vi "Create Cp plot.vi"(0 "Pressures in (cols = sensor, rows = time)":sgl[][](array[numeric])) -> (1 "Cp against x/c":cluster{"x/c flap (sorted)":sgl[], sgl[]}[](graph), 2 "Pdyn ref (Pa)":sgl)   [LabVIEW 2015]
panel:
  in  "Sensor index (sorted), cylinder":i32[](array[numeric])=[0, 1, 2, 3, 4, 5, 6, 7, 8, 9, 10, 11, 12, 13, 14, 15, 16, 17, 18, 19]
  in  "Pdyn ref sensor no.":i32=32
  in  "x/c cylinder (sorted)":sgl[](array[numeric])=[0.9659258, 0.8660254, 0.70710677, 0.5, 0.25881904, -0.25881904, -0.5, -0.70710677, -0.8660254, -0.9659258, -0.9659258, -0.8660254, -0.70710677, -0.5, -0.25881904, 0.25881904, 0.5, 0.70710677, 0.8660254, 0.9659258]
  # "Manually input and make default"
  # "Data sorted by winding no."
  # "Manually paste in data and then make default values"
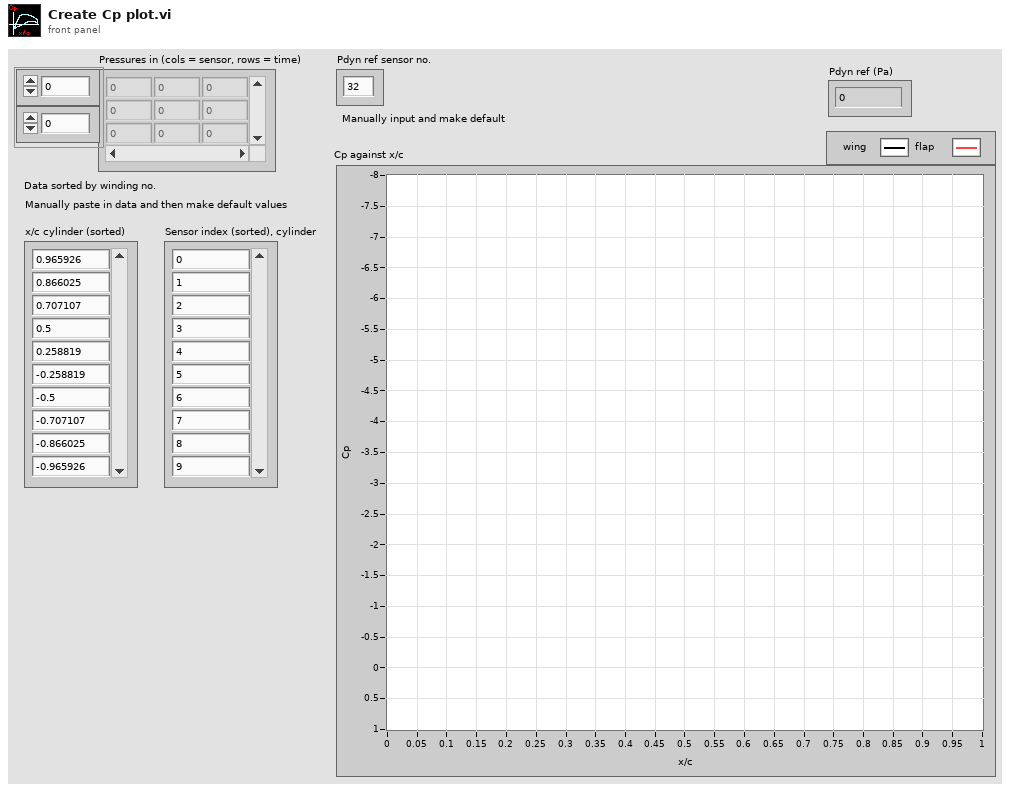
[diagram p1: front panel]
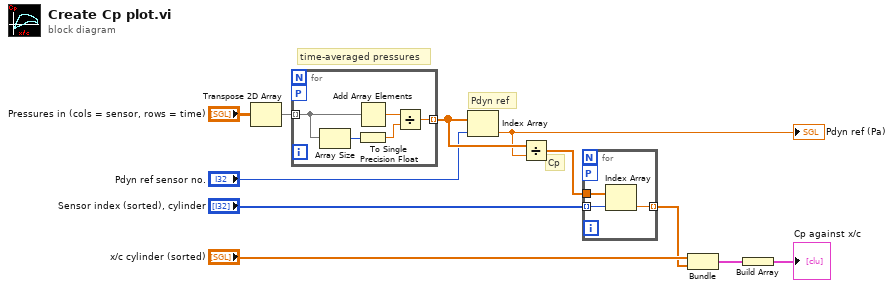
[diagram p0: block diagram]
diagram:
  # "Cp"
  # "Pdyn ref"
  # "time-averaged pressures"
  n1 = Transpose 2D Array(2D array="Pressures in (cols = sensor, rows = time)") -> (transposed array=w5:sgl[][])
  n2 = for {
    tunnel: w5 -> [w16] mode=indexing
    tunnel: [w12] -> w10 mode=indexing
    workers-P: _ -> [_]
    n3 = Array Size(array=w16) -> (size(s)=w14:i32)
    n4 = Add Array Elements(numeric array=w16) -> (sum=w15:sgl)
    n5 = To Single Precision Float(number=w14) -> (single precision float=w13:sgl)
    n6 = Divide(x=w15, y=w13) -> (x/y=w12:sgl)
  }
  n7 = Index Array(array=w10, index="Pdyn ref sensor no.") -> (element=w9:sgl)
  "Pdyn ref (Pa)" <- w9
  n8 = Divide(x=w10, y=w9) -> (x/y=w1:sgl[])
  n9 = for {
    tunnel: w1 -> [w19]
    tunnel: "Sensor index (sorted), cylinder" -> [w18] mode=indexing
    tunnel: [w17] -> w2 mode=indexing
    workers-P: _ -> [_]
    n10 = Index Array(array=w19, index=w18) -> (element=w17:sgl)
  }
  n11 = Bundle("x/c cylinder (sorted)"="x/c cylinder (sorted)", w2) -> (w6:cluster{"x/c cylinder (sorted)":sgl[], sgl[]})  [unwired: 1 in]
  n12 = Build Array(w6) -> (→"Cp against x/c":cluster{"x/c cylinder (sorted)":sgl[], sgl[]}[])
